vi "QAM2.vi"() -> ()   [LabVIEW 2019]
uses:
  <vilib>/addons/Modulation/Analog/support/mod_Set Error Source.vi
  <vilib>/addons/Modulation/Digital/Support/Common/Validators/mod_AWGN Validate.vi
  <vilib>/addons/Modulation/Digital/Impairments/subVIs/mod_createSeeds.vi
  <vilib>/addons/Modulation/Digital/Support/Common/Validators/mod_Validate Samples Per Symbol.vi
  <vilib>/addons/Modulation/Analog/support/Validators/mod_Validate Complex Waveform.vi
  <vilib>/addons/Modulation/Analog/support/Validators/mod_WFErrorHandler.vi
  <vilib>/addons/Modulation/Digital/General/MT Generate QAM System Parameters(M).vi
  <vilib>/addons/Modulation/Digital/Support/Common/Validators/mod_Generate Filter Coefficients Validate.vi
  <vilib>/addons/Modulation/Digital/General/subVIs/mod_Generate Filter Coefficients.vi
  <vilib>/addons/Modulation/Digital/General/subVIs/mod_Generate Bits PN Sequence.vi
  <vilib>/Analysis/1siggen.llb/Gaussian White Noise (obs 90).vi
  <vilib>/addons/Modulation/Analog/MT Upconvert Baseband (Real).vi
  <vilib>/express/express analysis/Spectral/Block/exnSpectralBlock spectral measurements RMS poly.vi
  <vilib>/express/express analysis/Spectral/Block/exnSpectralBlock spectral measurements RMS DDT.vi
  <vilib>/express/express analysis/Spectral/XNode/ExpressSpectralMeasurementsBlockNode.xnode
  <vilib>/addons/Modulation/niDMT.lvlib
  <vilib>/addons/Modulation/niAMT.lvlib
panel:
  in  "stop":bool
  in  "Message to send":string
  in  "Tab Control":T1(tab)
  out "Bassband Waveform 1":cluster{"t0":dbl, "dt":dbl, "Y":dbl[]}(graph)
  out "Bassband Waveform 2":cluster{"t0":dbl, "dt":dbl, "Y":dbl[]}(graph)
  out "Passband Waveform":waveform(dbl)(graph)
  out "Constellation Graph":T2(graph)
  out "FFT (RMS)":dynamicdata(graph)
  in  "Add Bit Padding":bool
  in  "carrier frequency (Hz)":dbl min=-0.5 max=0.5 format="%.0p"
  in  "Eb/N0 (10 dB)":dbl=10.0
  out "String Match":bool
  out "Demodulated String":string
  in  "autoscale":bool
  in  "Reset":bool
  in  "symbol rate (Hz)":dbl=1.0 format="%.0p"
  in  "pulse shaping filter (none)":T3(ring)
  in  "M-QAM (16)":u16(ring) items=["16"=16, "8"=8, "4"=4]
  # "QAM"
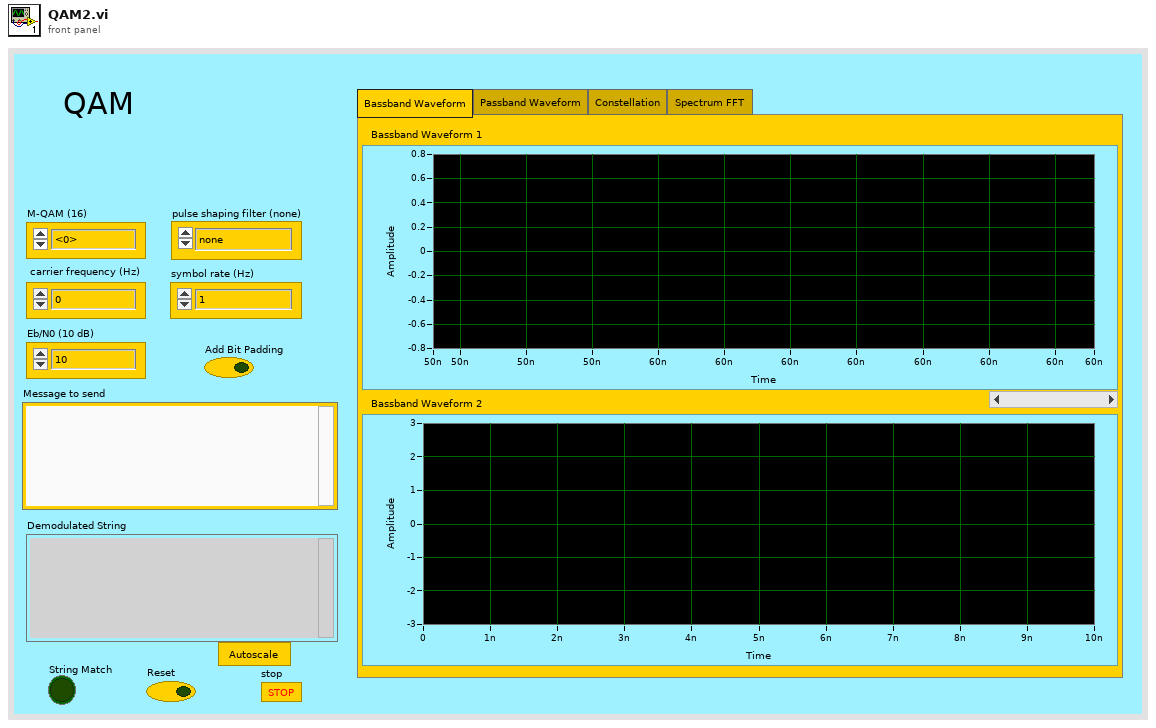
[diagram p1: front panel]
types:
  T1 = enum32{"Bassband Waveform", "Passband Waveform", "Constellation", "Spectrum FFT "}
  T2 = cluster{"Decimated Array":dbl[], "Decimated Array":dbl[]}[]
  T3 = enum16{"none", "Raised Cosine", "Root Raised Cos", "Gaussian"}
  T4 = enum16{"FSK", "PSK", "QAM", "MSK", "PAM", "ASK", "CPM"}
  T5 = cluster{"averaging mode":u16, "weighting mode":u16, "number of averages":u32}
  T6 = cluster{"dB On (F)":bool, "unwrap phase (F)":bool, "convert to degree (F)":bool}
  T7 = cluster{"samples per symbol (16)":i32, "symbol map":cdb[]}
  T8 = typedef "niAMT.lvlib/Complex Data Waveform.ctl" = cluster{"t0":dbl, "dt":dbl, "Y":cdb[]}
  T9 = cluster{"constellation":dbl[], "oversampled data":dbl[]}[]
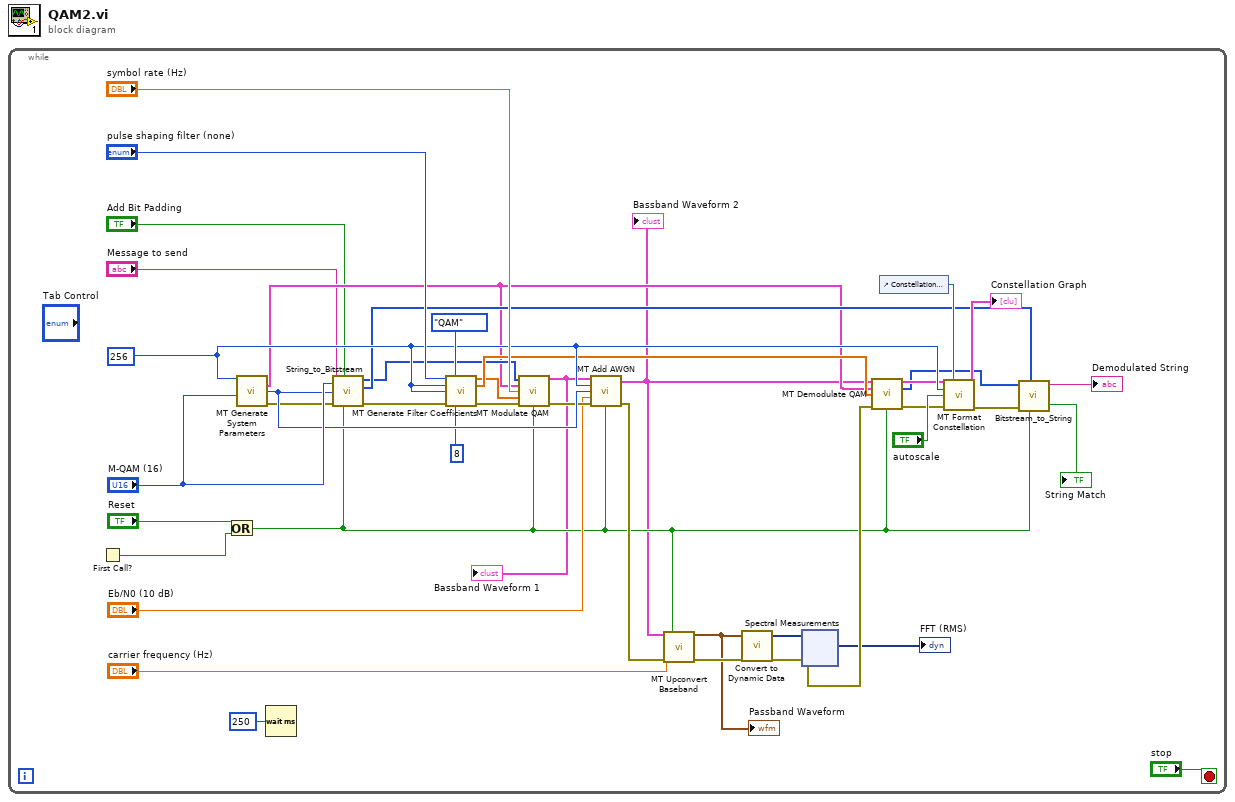
[diagram p0: block diagram]
diagram:
  n1 = while {
    stop <- "stop" stop-if-true
    w19 = 256 ("samples per symbol (16)")
    n2 = First Call?() -> (First Call?: T/F=w29:bool)
    n3 = Or(x="Reset", y=w29) -> (x .or. y?=w16:bool)
    n4 = call-poly <vilib>:"MT Generate System Parameters.vi"("samples per symbol (16)"=w19, "M-QAM (16)"="M-QAM (16)") -> ("QAM system parameters"=w10:T7, "bits per symbol"=w39:i32, "error out"=w34:errorcluster)  [unwired: 11 in]
    n5 = Wait (ms)(milliseconds to wait=u32 250) -> ()  [unwired: 1 out]
    n6 = call "String_to_Bitstream.vi"("Reset"=w16, "Add Bit Padding"="Add Bit Padding", "error in (no error)"=w34, "Guard Bits to Add"=w39, "M-ary (16)"="M-QAM (16)", "InputStrig"="Message to send") -> ("error out"=w33:errorcluster, "Character Array"=w12:u8[], "Bitstream (with Guard Bits)"=w11:i8[])  [unwired: 2 out]
    n7 = call <vilib>:"MT Generate Filter Coefficients.vi"("pulse shaping filter (none)"="pulse shaping filter (none)", "modulation type"=T4."QAM", "pulse shaping samples per symbol (16)"=w19, "matched samples per symbol (16)"=w19, "error in (no error)"=w33, "filter length (symbols)"=8) -> ("pulse shaping filter coefficients"=w14:dbl[], "matched filter coefficients"=w15:dbl[], "error out"=w32:errorcluster)  [unwired: 7 in]
    n8 = call <vilib>:"MT Modulate QAM.vi"("input bit stream"=w11, "QAM system parameters"=w10, "symbol rate (Hz)"="symbol rate (Hz)", "pulse shaping filter coefficients"=w14, "error in (no error)"=w32, "reset? (T)"=w16) -> ("output complex waveform"=w9:T8, "error out"=w31:errorcluster)  [unwired: 7 in, 1 out]
    "Bassband Waveform 1" <- w9
    n9 = call <vilib>:"MT Add AWGN.vi"("input complex waveform"=w9, "samples per symbol (16)"=w19, "bits per symbol (1)"=w39, "Eb/N0 (10 dB)"="Eb/N0 (10 dB)", "error in (no error)"=w31, "reset? (T)"=w16) -> ("output complex waveform"=w8:T8, "error out"=w27:errorcluster)  [unwired: 7 in, 1 out]
    "Bassband Waveform 2" <- w8
    n10 = call-poly <vilib>:"MT Upconvert Baseband.vi"("baseband waveform (complex)"=w8, "reset? (F)"=w16, "carrier frequency (Hz)"="carrier frequency (Hz)", "error in (no error)"=w27) -> ("passband waveform"=w4:waveform(dbl), "error out"=w25:errorcluster)  [unwired: 10 in]
    "Passband Waveform" <- w4
    n11 = call "Convert to Dynamic Data"("Waveform"=w4) -> ("Dynamic Data Type"=w26:dynamicdata)  [unwired: 3 in]
    n12 = xnode "Spectral Measurements"("Signals"=w26, "error in (no error)"=w25) -> ("FFT - (RMS)"=→"FFT (RMS)":dynamicdata, "error out"=w24:errorcluster)  [unwired: 1 out]
    n13 = call <vilib>:"MT Demodulate QAM.vi"("input complex waveform"=w8, "QAM system parameters"=w10, "matched filter coefficients"=w15, "error in (no error)"=w24, "reset? (T)"=w16) -> ("recovered complex waveform"=w13:T8, "output bit stream"=w7:i8[], "error out"=w23:errorcluster)  [unwired: 6 in, 2 out]
    n14 = control-ref of="Constellation Graph"() -> (w42:refnum<vi>)
    n15 = call <vilib>:"MT Format Constellation.vi"("waveform"=w13, "constellation reference"=w42, "samples per symbol"=w19, "autoscale"="autoscale", "error in (no error)"=w23) -> ("constellation graph"=→"Constellation Graph":T9, "error out"=w22:errorcluster)  [unwired: 9 out]
    n16 = call "Bitstream_to_String.vi"("Reset"=w16, "Character Array"=w12, "error in (no error)"=w22, "Bit Array"=w7) -> ("Demodulated String"=→"Demodulated String":string, "Match Found?"=→"String Match":bool)  [unwired: 2 in, 4 out]
  }
